vi "Limit trigger fgv.vi"(7 "Reset":bool, 8 "error in (no error)":errorcluster, 11 "Set":bool) -> (0 "error out":errorcluster, 3 "Limit trigger":bool)   [LabVIEW 2016]
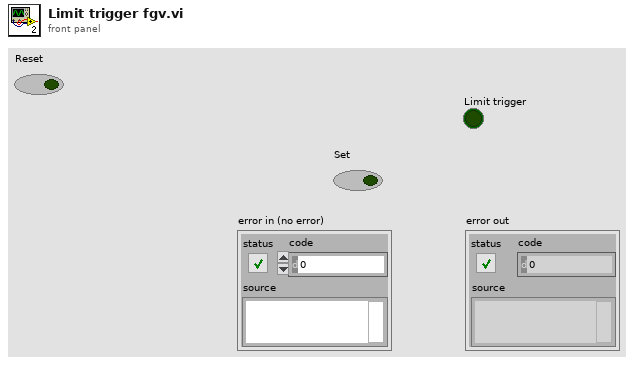
[diagram p1: front panel]
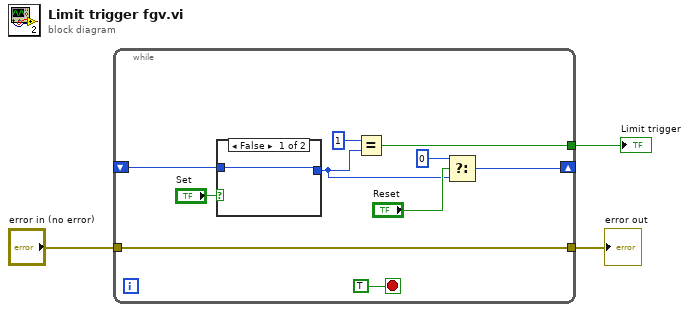
[diagram p0: block diagram]
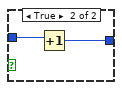
[diagram p2: hidden frame]
diagram:
  n1 = while {
    shift-right: [w4] -> _
    shift-left: _ -> [w12]
    tunnel: "error in (no error)" -> [w9]
    tunnel: [w9] -> w2
    tunnel: [w8] -> w1
    stop <- TRUE stop-if-true
    n2 = case shown="False" "Set" {
      tunnel: w12 -> [w14 w16]
      tunnel: [w14 w15] -> w5
      frame False {
      }
      frame True {
        n3 = Increment(x=w16) -> (x+1=w15:i32)
      }
    }
    n4 = Equal?(x=1, y=w5) -> (x = y?=w8:bool)
    n5 = Select(t=0, s="Reset", f=w5) -> (s? t:f=w4:i32)
  }
  "Limit trigger" <- w1
  "error out" <- w2
